vi "Motion@AddPath__Parameter.vi"(1 "ParamterIn":string) -> (0 "ParamterOut":string)   [LabVIEW 2019]
panel:
  in  "PointName":string(combo)
  in  "Speed":string(combo)
  in  "MotorName":string(combo)
  in  "Confirm":bool
  # "Motor@GoPoint/GoPallet/AddPath $Motor,$Speed,$Point"
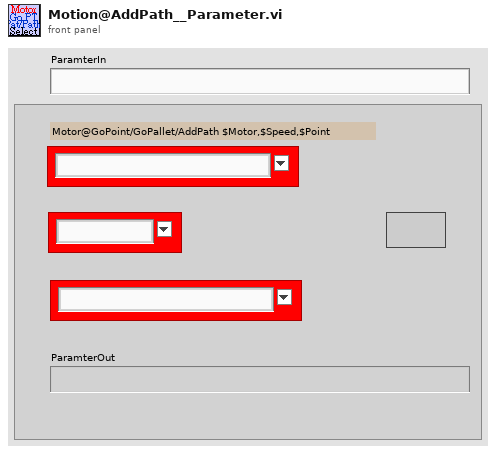
[diagram p1: front panel]
types:
  T1 = enum16{"Get", "UpdatePointS", "Init", "UpdateIndex", "GetCurrent&Index+1", "GetWithIndex", "ChkLast", "GetCurrent"}
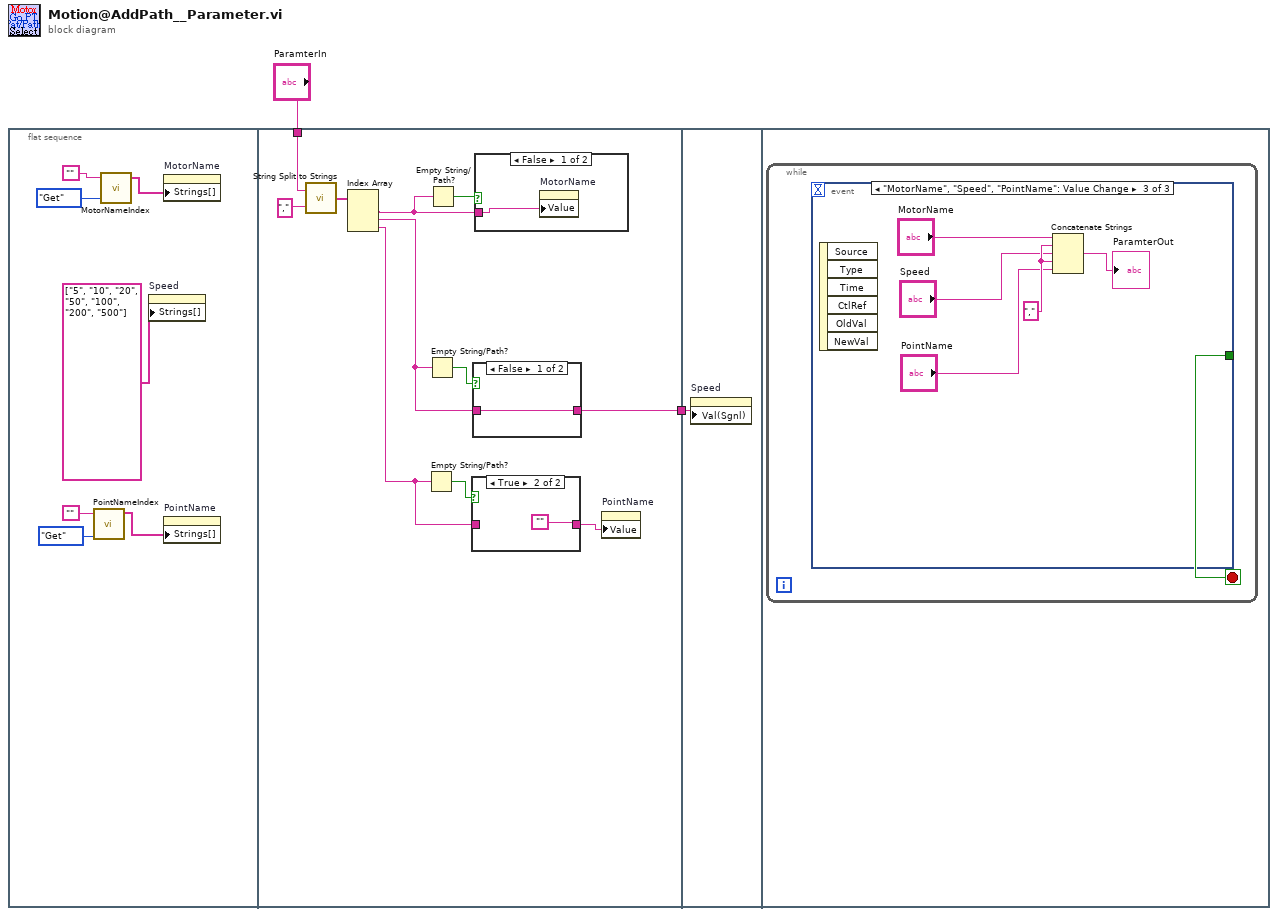
[diagram p0: block diagram]
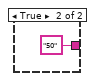
[diagram p3: hidden frame]
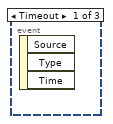
[diagram p5: hidden frame]
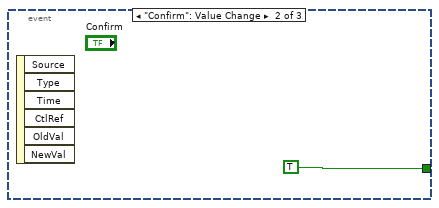
[diagram p6: hidden frame]
diagram:
  n1 = flat-sequence {
    tunnel: "ParamterIn" -> [w16]
    tunnel: [w11] -> w1
    tunnel: w1 -> [w26]
    frame #0 {
      n2 = call "PointNameIndex.vi"("OP"=T1."Get", "PointName"="") -> ("PointNameList"=w3:string[])  [unwired: 4 in, 5 out]
      n3 = call "MotorNameIndex.vi"("OP"=enum16{"Get", "Update", "Init"}."Get", "MotorName"="") -> ("MotorList"=w7:string[])  [unwired: 1 in, 2 out]
      n4 = property on="Speed" class="CmbBox"("Strings[]"=string[] ["5", "10", "20", "50", "100", "200", "500"] ("Strings []")) -> ()  [unwired: 2 in, 2 out]
      n5 = property on="MotorName" class="CmbBox"("Strings[]"=w7) -> ()  [unwired: 2 in, 2 out]
      n6 = property on="PointName" class="CmbBox"("Strings[]"=w3) -> ()  [unwired: 2 in, 2 out]
    }
    frame #1 {
      n7 = call "String Split to Strings.vi"("search string/char (-)"=",", "String"=w16) -> ("Array"=w18:string[])
      n8 = Index Array(array=w18) -> (element #1=w15:string, element #2=w14:string, element #3=w12:string)  [unwired: 3 in]
      n9 = Empty String/Path?(string/path=w12) -> (empty?=w13:bool)
      n10 = Empty String/Path?(string/path=w14) -> (empty?=w19:bool)
      n11 = Empty String/Path?(string/path=w15) -> (empty?=w20:bool)
      n12 = case shown="True" w13 {
        tunnel: [w21 ""] -> w10
        tunnel: w12 -> [w21 _]
        frame False {
        }
        frame True {
        }
      }
      n13 = case shown="False" w19 {
        tunnel: [w23 "50" ("ParamterIn")] -> w11
        tunnel: w14 -> [w23 _]
        frame False {
        }
        frame True {
        }
      }
      n14 = case shown="False" w20 {
        tunnel: w15 -> [w25 _]
        frame False {
          n15 = property on="MotorName" class="CmbBox"("Value"=w25) -> ()  [unwired: 2 in, 2 out]
        }
        frame True {
        }
      }
      n16 = property on="PointName" class="CmbBox"("Value"=w10) -> ()  [unwired: 2 in, 2 out]
    }
    frame #2 {
      n17 = property on="Speed" class="CmbBox"("Val(Sgnl)"=w26) -> ()  [unwired: 2 in, 2 out]
    }
    frame #3 {
      n18 = while {
        stop <- w27 stop-if-true
        n19 = event shown="[2] \"MotorName\", \"Speed\", \"PointName\": Value Change" {
          selector: _ -> [_ _ _]
          dyn-events: _ -> [_ _ _]
          timeout: _ -> [_ _ _]
          tunnel: [_ TRUE _] -> w27
          event Timeout {
            n20 = event-data() -> ()  [unwired: 1 in, 3 out]
          }
          event "Confirm": Value Change {
            n21 = event-data() -> ()  [unwired: 1 in, 6 out]
          }
          event "MotorName", "Speed", "PointName": Value Change {
            w31 = "," ("string")
            n22 = event-data() -> ()  [unwired: 1 in, 6 out]
            n23 = Concatenate Strings("MotorName", w31, "Speed", w31, "PointName") -> (→"ParamterOut":string)
          }
        }
      }
    }
  }
